vi "Main.vi"() -> ()   [LabVIEW 2012]
doc: "Fill in description for your main VI here."
uses:
  Data type A.ctl
  Data type B.ctl
  <vilib>/Platform/TimedLoop/XDataNode/timing_clust.ctl
  <vilib>/Platform/TimedLoop/XDataNode/nitl_modes.ctl
  <vilib>/Platform/TimedLoop/XDataNode/wakeup.ctl
  <vilib>/Platform/TimedLoop/XDataNode/XDataNode.xnode
  <vilib>/Platform/TimedLoop/XDataNode/XDNodeRunTimeDep.lvlib
panel:
  in  "stop":bool
  out "error out":errorcluster
  in  "error in (no error)":errorcluster
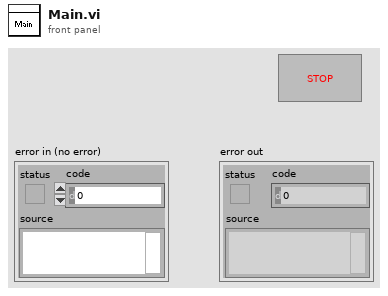
[diagram p1: front panel]
types:
  T1 = typedef "Data type B.ctl" = cluster{"Numeric":dbl, "Boolean":bool}
  T2 = typedef "Data type A.ctl" = dbl
  T3 = typedef "XDNodeRunTimeDep.lvlib/timing_clust.ctl" = cluster{"Expected End [f-1]":u64, "Actual End [f-1]":u64, "Finished Late? [f-1]":bool, "Expected End [i-1]":u64, "Actual End [i-1]":u64, "Finished Late? [i-1]":bool, "Expected Start [i]":u64, "Actual Start [i]":u64, "Expected Start [f]":u64, "Actual Start [f]":u64, "Source Name":string, "Structure Name":string, "Period":i64, "Deadline":i64, "Offset":i64, "Start":i64, "Priority":i32, "Timeout":i32, "Mode":T4, "Wakeup Reason":T5, "Error":errorcluster, "Source Type":string, "Secondary Source Type":string, "Global End Time":u64, "Global Start Time":u64, "Frame Duration":u64, "Iteration Duration":u64, "Assigned CPU":i32, "I/O Scan Engine Mode":u32}
  T4 = typedef "XDNodeRunTimeDep.lvlib/nitl_modes.ctl" = enum32{"No Change", "Process missed periods, maintain original phase", "Discard missed periods, maintain original phase", "Process missed periods, ignore original phase", "Discard missed periods, ignore original phase"}
  T5 = typedef "XDNodeRunTimeDep.lvlib/wakeup.ctl" = enum32{"Normal", "Aborted", "Asynchronous wakeup", "Timing source error", "Timed loop error", "Timeout"}
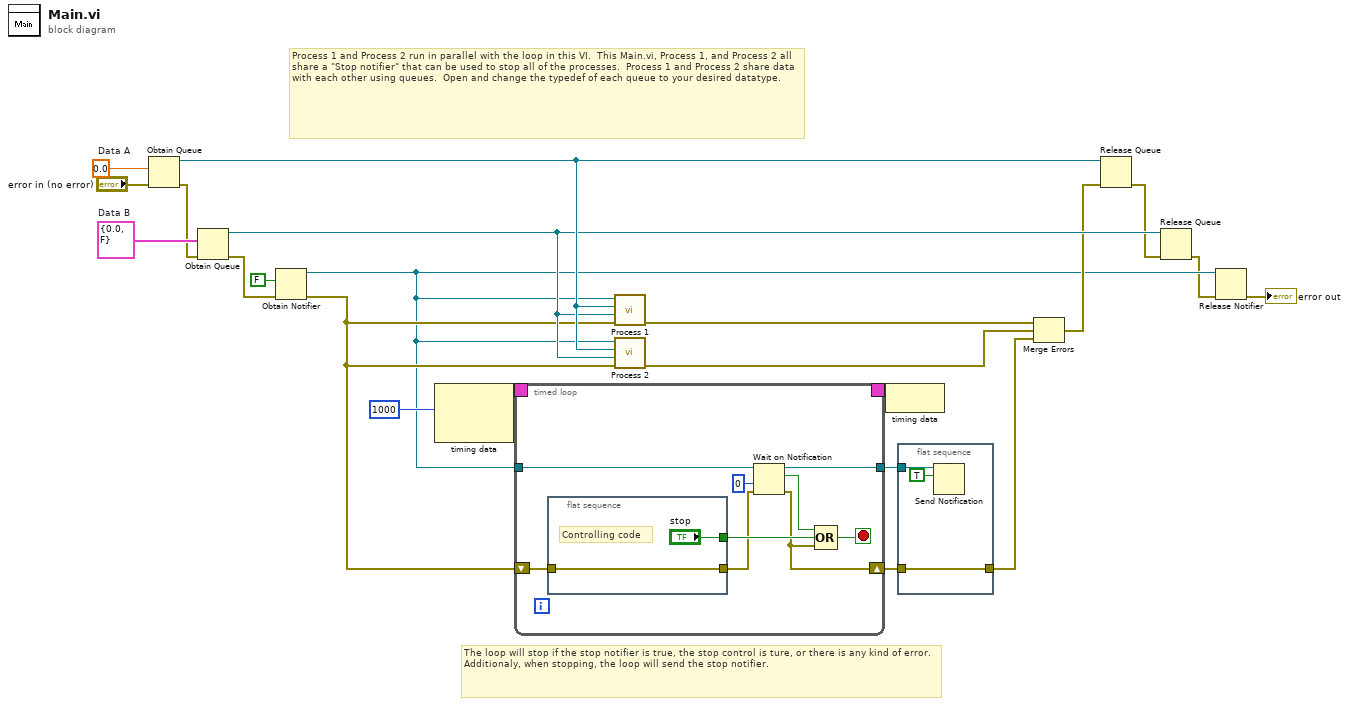
[diagram p0: block diagram]
diagram:
  w19 = T1 {"Numeric"=0.0, "Boolean"=FALSE}  # Data B
  w20 = T2 0.0  # Data A
  # "The loop will stop if the stop notifier is true, the stop control is ture, or there is any kind of error.\nAdditionaly, when stopping, the loop will send the stop notifier."
  # "Process 1 and Process 2 run in parallel with the loop in this VI.  This Main.vi, Process 1, and Process 2 all share a \"Stop notifier\" that can be used to stop all of the processes.  Process 1 and Process 2 share data with each other using queues.  Open and change the typedef of each queue to your desired datatype."
  n1 = Obtain Queue(element data type=w20, error in (no error)="error in (no error)") -> (queue out=w15:refnum<queue>, error out=w14:errorcluster)  [unwired: 3 in, 1 out]
  n2 = Obtain Queue(element data type=w19, error in (no error)=w14) -> (queue out=w13:refnum<queue>, error out=w11:errorcluster)  [unwired: 3 in, 1 out]
  n3 = Obtain Notifier(notification data type=FALSE ("Stop"), error in (no error)=w11) -> (notifier out=w4:refnum<notifier>, error out=w10:errorcluster)  [unwired: 2 in, 1 out]
  n4 = node-c288(i64 1000 ("Period")) -> (w22:T3)  [unwired: 1 in]
  n5 = timed-loop {
    timing: w22 -> [_]
    timing-out: [_] -> w21
    tunnel: w4 -> [w30]
    shift-right: [w24] -> w9
    shift-left: w10 -> [w27]
    tunnel: [w26] -> w16
    stop <- w28 stop-if-true
    n6 = flat-sequence {
      tunnel: w27 -> [w33]
      tunnel: [w33] -> w23
      tunnel: ["stop"] -> w25
      frame #0 {
        # "Controlling code"
      }
    }
    n7 = Wait on Notification(notifier=w30, timeout in ms (-1)=0, error in (no error)=w23) -> (notifier out=w26:refnum<notifier>, notification=w29:bool, error out=w24:errorcluster)  [unwired: 1 in, 1 out]
    n8 = Compound Arithmetic op=OR(w29, w25, w24) -> (w28:bool)
  }
  n9 = call "Process 1.vi"("error in (no error)"=w10, "Data B queue"=w13, "Data A queue"=w15, "Stop notifier"=w4) -> ("error out"=w7:errorcluster)  [unwired: 7 in]
  n10 = call "Process 2.vi"("error in (no error)"=w10, "Data B queue"=w13, "Data A queue"=w15, "Stop notifier"=w4) -> ("error out"=w6:errorcluster)  [unwired: 7 in]
  n11 = node-c288(w21) -> ()
  n12 = flat-sequence {
    tunnel: w16 -> [w37]
    tunnel: w9 -> [w36]
    tunnel: [w36] -> w8
    frame #0 {
      n13 = Send Notification(notification=TRUE, notifier=w37) -> ()  [unwired: 1 in, 2 out]
    }
  }
  n14 = Merge Errors(w7, w6, w8) -> (w5:errorcluster)
  n15 = Release Queue(queue=w15, error in (no error)=w5) -> (error out=w12:errorcluster)  [unwired: 1 in, 2 out]
  n16 = Release Queue(queue=w13, error in (no error)=w12) -> (error out=w3:errorcluster)  [unwired: 1 in, 2 out]
  n17 = Release Notifier(notifier=w4, error in (no error)=w3) -> (error out=→"error out":errorcluster)  [unwired: 1 in, 2 out]
